vi "WPI_AnalogModuleGetAverageValue.vi"(8 "error in (no error)":errorcluster, 10 "Channel":T2=enum."AI 1", 11 "AnalogModuleDevRef":T1) -> (0 "error out":errorcluster, 2 "AveragedValue":i32, 3 "AnalogModuleDevRef":T1)   [LabVIEW 2017]
doc: "This software is licensed. Open the labview\\readme\\WPI Robotics Library Open Source License.txt file for more information."
uses:
  <vilib>/Rock Robotics/SystemInterfaces/AI/FPGA_AIChannel.ctl
  <vilib>/Rock Robotics/WPI/AnalogModule/WPI_AnalogModuleDevStatus.ctl
  <vilib>/Rock Robotics/SystemInterfaces/System/FPGA_SystemGet.vi
  <vilib>/Rock Robotics/SystemInterfaces/AI/FPGA_ReadAI.vi
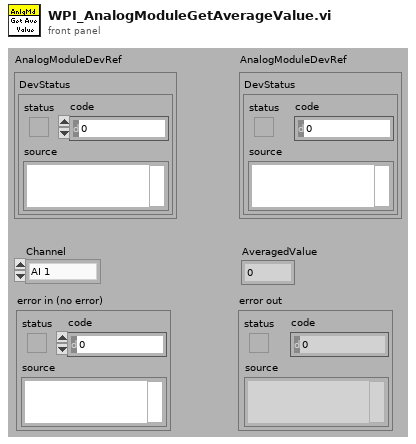
[diagram p1: front panel]
types:
  T1 = typedef "WPI_AnalogModuleDevStatus.ctl" = cluster{"DevStatus":errorcluster}
  T2 = typedef "FPGA_AIChannel.ctl" = enum8{"AI 0", "AI 1", "AI 2", "AI 3", "AI MXP 0", "AI MXP 1", "AI MXP 2", "AI MXP 3", "Invalid"}
  T3 = typedef "FPGA_AIDevRef.ctl" = cluster{"DevStatus":errorcluster}
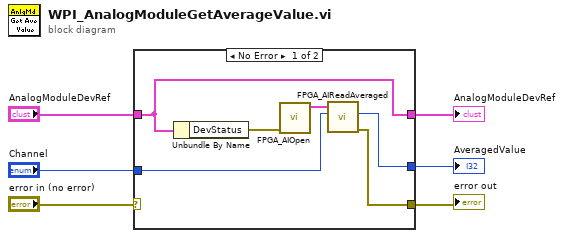
[diagram p0: block diagram]
diagram:
  n1 = case shown="No Error" "error in (no error)" {
    selector: "error in (no error)" -> [_ w14]
    tunnel: "AnalogModuleDevRef" -> [w7 w13]
    tunnel: [w7 w13] -> w5
    tunnel: "Channel" -> [w10 _]
    tunnel: [w9 _] -> w3
    tunnel: [w8 w14] -> w1
    frame No Error {
      n2 = Unbundle By Name(w7) -> ("DevStatus"=w12:errorcluster)
      n3 = call <vilib>:"FPGA_AIOpen.vi"("error in (no error)"=w12) -> ("AI Reference out"=w11:T3)  [unwired: 2 in, 8 out]
      n4 = call <vilib>:"FPGA_AIReadAveraged.vi"("Channel"=w10, "AI Reference in"=w11) -> ("error out"=w8:errorcluster, "Averaged"=w9:i32)  [unwired: 1 in, 7 out]
    }
    frame Error {
    }
  }
  "AnalogModuleDevRef" <- w5
  "AveragedValue" <- w3
  "error out" <- w1
